vi "Database.Handler.SendData.vi"(8 "error in":errorcluster, 11 "Data in":T1) -> (0 "error out":errorcluster, 3 "Data out":T1)   [LabVIEW 2016]
doc: "Write test results (measurement values) to proda database\n\nWabco 2017 All right reserved\nAuthor: maciej.szupienko@wabco-auto.com"
uses:
  Database.Handler.Data.ctl
  Database.Handler.Data.Status.ctl
  Database.Handler.Data.Sets.ctl
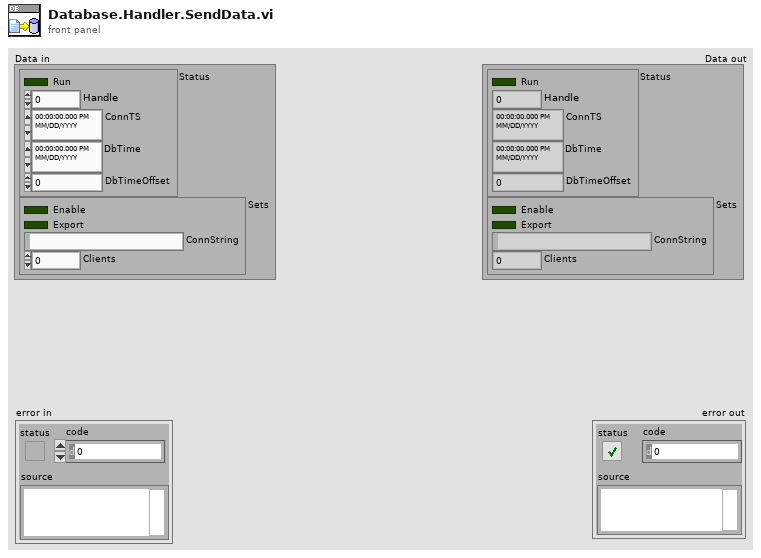
[diagram p1: front panel]
types:
  T1 = typedef "Database.Handler.Data.ctl" = cluster{"Status":T2, "Sets":T3}
  T2 = typedef "Database.Handler.Data.Status.ctl" = cluster{"Run":bool, "Handle":i32, "ConnTS":timestamp, "DbTime":timestamp, "DbTimeOffset":dbl}
  T3 = typedef "Database.Handler.Data.Sets.ctl" = cluster{"Enable":bool, "Export":bool, "ConnString":string, "Clients":i32}
  T4 = typedef "ProdaNG.ProductComponent.ctl" = cluster{"product_wabcoNumber":string, "product_serialNumber":string, "component_wabcoNumber":string, "component_serialNumber":string, "pressStepResultId":string, "qty":i32, "level":i32}
  T5 = typedef "Cache.TestSteps.Fglb.ResultData.ctl" = cluster{"File":path, "Ref":string, "Serial":string, "Pr":T6, "PSr":T7, "TSr":cluster{"TSr":T8, "TVr":T9[]}[]}
  T6 = typedef "ProdaNG.ProcessResult.ctl" = cluster{"c_id":string, "productId":string, "processId":i32, "statusId":i32, "startTime":string, "endTime":string}
  T7 = typedef "ProdaNG.ProcessStepResult.ctl" = cluster{"c_id":string, "processResultId":string, "processStepId":i32, "statusId":i32, "operatorId":i32, "startTime":string, "endTime":string}
  T8 = typedef "ProdaNG.TestStepResult.ctl" = cluster{"c_id":string, "processStepResultId":string, "testStepId":i32, "statusId":i32}
  T9 = typedef "ProdaNG.TestValueResult.ctl" = cluster{"c_id":string, "testStepResultId":string, "testValueId":i32, "result":dbl, "statusId":i32, "contentId":string}
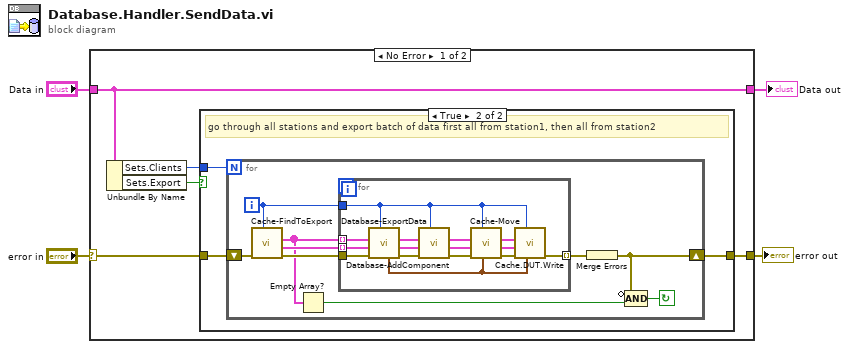
[diagram p0: block diagram]
diagram:
  n1 = case shown="No Error" "error in" {
    selector: "error in" -> [w9 w34]
    tunnel: [w8 w34] -> w4
    tunnel: "Data in" -> [w6 w33]
    tunnel: [w6 w33] -> w1
    frame No Error {
      n2 = Unbundle By Name(w6) -> ("Sets.Clients"=w5:i32, "Sets.Export"=w7:bool)
      n3 = case shown="True" w7 {
        tunnel: w9 -> [w10 w13]
        tunnel: [w10 w12] -> w8
        tunnel: w5 -> [_ w11]
        frame False {
        }
        frame True {
          # "go through all stations and export batch of data first all from station1, then all from station2"
          n4 = for {
            N: w11 -> [_]
            shift-right: [w14] -> w12
            shift-left: w13 -> [w19]
            i -> [w18]
            stop <- w20 continue-if-true
            n5 = call "Cache-FindToExport.vi"("Idx"=w18, "error in"=w19) -> ("error out"=w17:errorcluster, "ProductComponent"=w16:T4[], "Results"=w15:T5[])  [unwired: 7 in]
            n6 = Empty Array?(array=w15) -> (empty?=w22:bool)
            n7 = for {
              tunnel: w17 -> [w29]
              tunnel: w18 -> [w31]
              tunnel: [w23] -> w21 mode=indexing
              tunnel: w15 -> [w28] mode=indexing
              tunnel: w16 -> [w27] mode=indexing
              n8 = call "Database-ExportData.vi"("Idx"=w31, "error in"=w29, "Result in"=w28) -> ("error out"=w32:errorcluster, "Result out"=w26:T5, "Export time"=w30:timestamp)  [unwired: 6 in]
              n9 = call "Database-AddComponent.vi"("Idx"=w31, "error in"=w32, "ProductComponent"=w27) -> ("error out"=w25:errorcluster)  [unwired: 8 in]
              n10 = call "Cache-Move.vi"("Time (now)"=w30, "Idx"=w31, "error in"=w25, "Result in"=w26) -> ("error out"=w24:errorcluster)  [unwired: 7 in]
              n11 = call "Cache.DUT.Write.vi"("Time (now)"=w30, "Idx"=w31, "error in (no error)"=w24, "ProductComponent"=w27, "Result in"=w26) -> ("error out"=w23:errorcluster)  [unwired: 6 in]
            }
            n12 = Merge Errors(w21) -> (w14:errorcluster)
            n13 = Compound Arithmetic op=AND(invert w14, w22) -> (w20:bool)
          }
        }
      }
    }
    frame Error {
    }
  }
  "error out" <- w4
  "Data out" <- w1
